vi "LVClass_CorrectionDataManager RemovePupilMask.vi"(0 "CorrectionDataManager in":refnum<class "CorrectionDataManager.lvclass">, 11 "error in (no error)":errorcluster) -> (4 "CorrectionDataManager out":refnum<class "CorrectionDataManager.lvclass">, 15 "error out":errorcluster)   [LabVIEW 2020, in "CorrectionDataManager.lvclass"]
doc: "Sets the greatest common pupil.\n\n--------------------------------------------------------------------------------\n\n<B>corrdata_managerIn </B> : CorrDataManager object.\n<B>corrdata_managerOut </B> : CorrDataManager object.\n<B>pupil </B> : User-defined greatest common pupil as a pointer on a pupil object.\n<B>ErrorIn </B> : Error\n<B>ErrorOut </B> : Error\n\n--------------------------------------------------------------------------------"
uses:
  CorrectionDataManager.lvclass
  CorrectionDataManager.lvclass/CorrectionDataManager.ctl
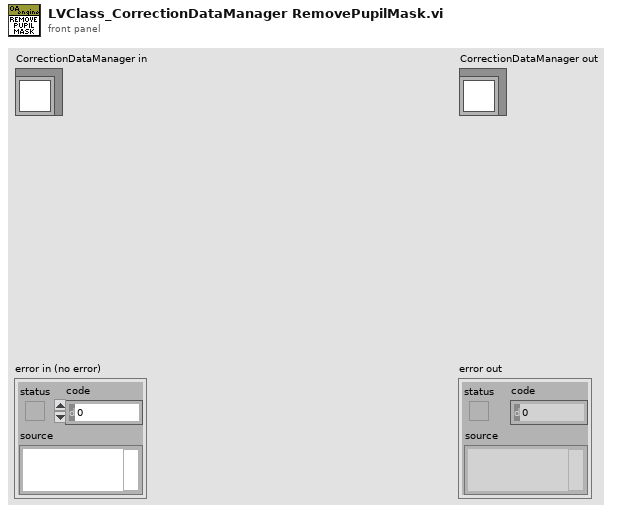
[diagram p1: front panel]
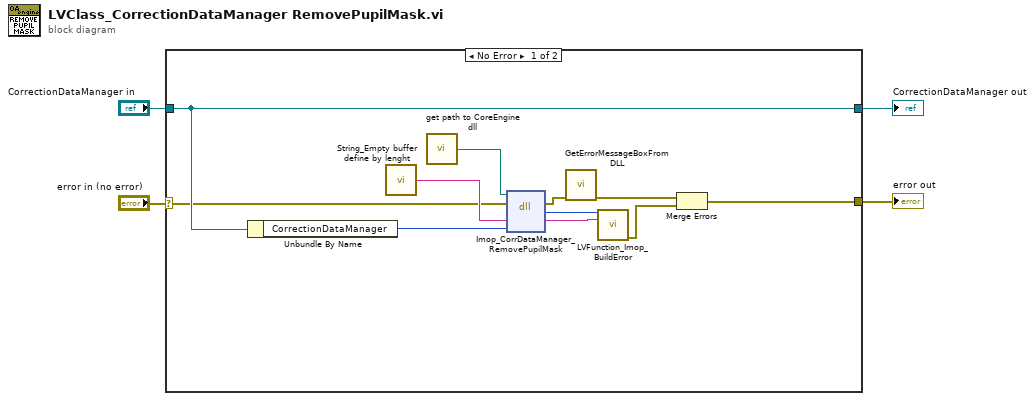
[diagram p0: block diagram]
diagram:
  n1 = case shown="No Error" "error in (no error)" {
    selector: "error in (no error)" -> [w5 w17]
    tunnel: [w6 w17] -> w2
    tunnel: [w8 w16] -> w1
    tunnel: "CorrectionDataManager in" -> [w8 w16]
    frame No Error {
      n2 = Unbundle By Name(w8) -> ("CorrectionDataManager"=w7:i32)
      n3 = call "String_Empty buffer define by lenght.vi"() -> ("Empty buffer"=w13:string)  [unwired: 1 in]
      n4 = call "get path to CoreEngine dll.vi"() -> ("path to c_interface_vc100.dll"=w9:path)  [unwired: 12 in, 3 out]
      n5 = dll-call lib="D:/FLE/0.Code/CoreEngine4_Suite/LV2011_interface/DLLs/c_interface_vc100.dll" fn="Imop_CorrDataManager_RemovePupilMask"(path in=w9, error in=w5, "message"=w13, "corrdata_manager"=w7) -> (error out=w12:errorcluster, "return type"=w15:i32, "message"=w14:string)  [unwired: 2 in, 1 out]
      n6 = call "GetErrorMessageBoxFromDLL.vi"("error IN"=w12) -> ("error OUT"=w11:errorcluster)  [unwired: 10 in]
      n7 = call "LVFunction_Imop_BuildError.vi"("code"=w15, "String to Prepend to source (\"\")"=w14) -> ("error out"=w10:errorcluster)  [unwired: 13 in]
      n8 = Merge Errors(w11, w10) -> (w6:errorcluster)
    }
    frame Error {
    }
  }
  "error out" <- w2
  "CorrectionDataManager out" <- w1
